vi "Call Chain (Single String).vi"() -> (0 "Call Chain":string)   [LabVIEW 2013]
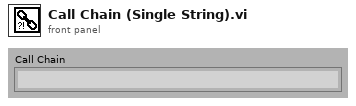
[diagram p1: front panel]
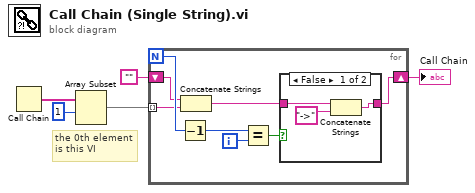
[diagram p0: block diagram]
diagram:
  # "the 0th element\nis this VI"
  n1 = Call Chain() -> (call chain=w3:string[])
  n2 = Array Subset(array=w3, index=1) -> (w5:string[])  [unwired: 1 in]
  n3 = for {
    N -> [w10]
    tunnel: w5 -> [w8] mode=indexing
    shift-right: [w6] -> w2
    shift-left: "" -> [w9]
    i -> [w7]
    n4 = Decrement(x=w10) -> (x-1=w13:i32)
    n5 = Concatenate Strings(w9, w8) -> (w11:string)
    n6 = Equal?(x=w13, y=w7) -> (x = y?=w12:bool)
    n7 = case shown="False" w12 {
      tunnel: w11 -> [w16 w17]
      tunnel: [w14 w17] -> w6
      frame False {
        n8 = Concatenate Strings(w16, "->" ("Substring")) -> (w14:string)
      }
      frame True {
      }
    }
  }
  "Call Chain" <- w2
